vi "Keep Last n Rows 2D.vi"(10 "Array":dbl[][](array[numeric]) format="%.3f", 11 "# Rows to Keep":i32=1) -> (2 "Last n Rows":dbl[][](array[numeric]) format="%.3f")   [LabVIEW 2019]
panel:
  # "Splits off the last n rows of a 2D array.  Used where you keep appending new data to the end of an array,\nand just want to keep the most recent n rows."
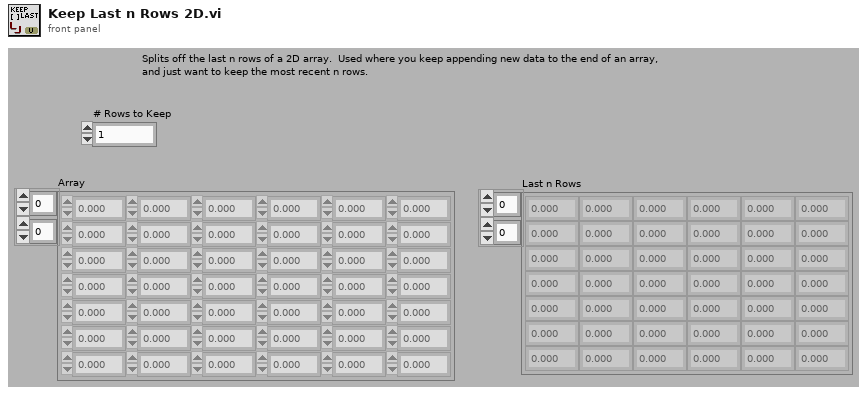
[diagram p1: front panel]
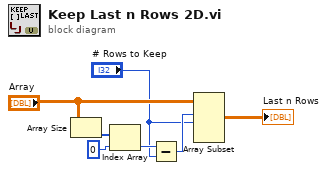
[diagram p0: block diagram]
diagram:
  n1 = Array Size(array="Array") -> (size(s)=w7:i32[])
  n2 = Index Array(array=w7, index=0) -> (element=w5:i32)
  n3 = Subtract(x=w5, y="# Rows to Keep") -> (x-y=w4:i32)
  n4 = Array Subset(array="Array", index (row)=w4, length (row)="# Rows to Keep") -> (→"Last n Rows":dbl[][])  [unwired: 2 in]
